vi "PP Template.vi"() -> ()   [LabVIEW 2011, in "Messenging.lvlib" / "PP Template.lvclass"]
uses:
  PP Template.lvclass
  Parallel Process.lvclass
  Interprocess Messenger/TextVarientMessage/MSG.lvclass
  Interprocess Messenger/Receiver/MGR (Receive type).lvclass
  ObserverRegister/ObserverRegistry.lvclass
  Interprocess Messenger/TextVarientMessage/Write (no data).vi
  Interprocess Messenger/TextVarientMessage/Write VarMessage.vi
  Interprocess Messenger/VarMessage/VarMessage.lvclass
  Interprocess Messenger/TextVarientMessage/Extract Text (static).vi
panel:
  out "date/time string":string
  in  "Startup Message":refnum<class "MSG.lvclass">
  # "QueueMessenger Based"
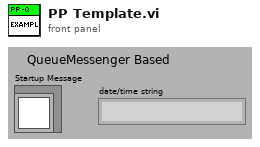
[diagram p1: front panel]
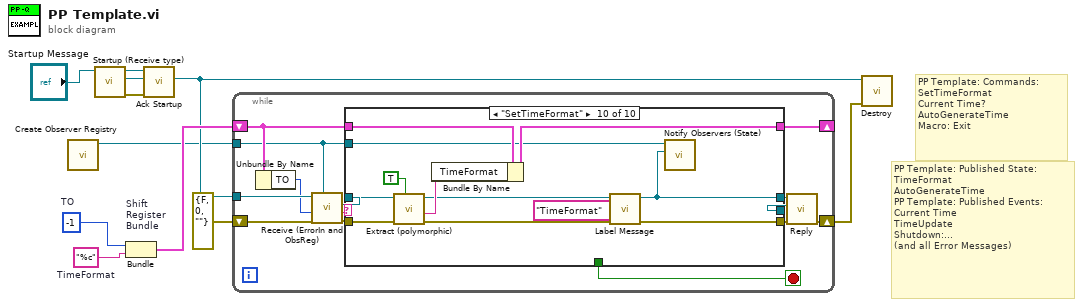
[diagram p0: block diagram]
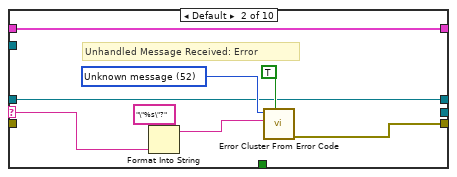
[diagram p3: hidden frame]
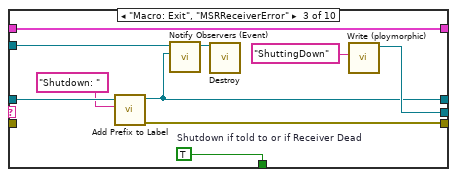
[diagram p4: hidden frame]
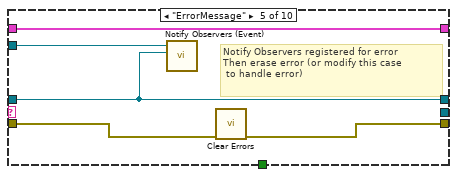
[diagram p6: hidden frame]
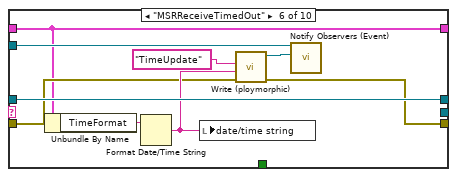
[diagram p7: hidden frame]
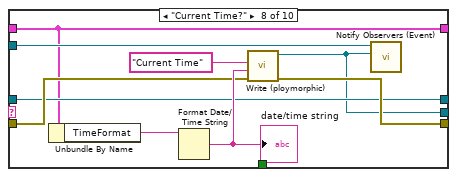
[diagram p9: hidden frame]
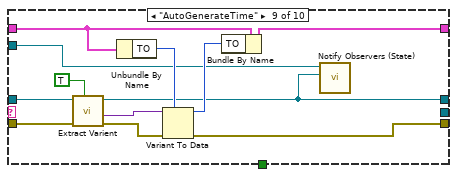
[diagram p10: hidden frame]
diagram:
  w3 = "%c"  # TimeFormat
  w8 = -1  # TO
  # "PP Template: Published State:\nTimeFormat\nAutoGenerateTime\nPP Template: Published Events:\nCurrent Time\nTimeUpdate\nShutdown:...\n(and all Error Messages)"
  # "PP Template: Commands:\nSetTimeFormat\nCurrent Time?\nAutoGenerateTime\nMacro: Exit"
  n1 = call "Create Observer Registry.vi"() -> ("ObsReg"=w2:refnum<class "ObserverRegistry.lvclass">)  [unwired: 1 in, 10 out]
  n2 = call "Startup (Receive type).vi"("Startup Message"="Startup Message") -> ("error out"=w5:errorcluster, "Command Messenger out"=w6:refnum<class "MGR (Receive type).lvclass">, "Starup Message"=w11:refnum<class "MSG.lvclass">)  [unwired: 1 in, 7 out]
  n3 = Bundle "Shift\nRegister\nBundle"("TO"=w8, "TimeFormat"=w3) -> (w7:cluster{"TO":i32, "TimeFormat":string})  [unwired: 1 out]
  n4 = call "Ack Startup.vi"("error in"=w5, "Command Messenger"=w6, "Starup Message"=w11) -> ("Command Messenger"=w4:refnum<class "MGR (Receive type).lvclass">)  [unwired: 3 in, 5 out]
  n5 = while {
    shift-right: [w23] -> w9
    shift-left: errorcluster {"status"=FALSE, "code"=0, "source"=""} ("error out") -> [w15]
    shift-right: [w20] -> _
    shift-left: w7 -> [w19]
    tunnel: w4 -> [w14]
    tunnel: w2 -> [w13]
    stop <- w21 stop-if-true
    n6 = Unbundle By Name(w19) -> ("TO"=w12:i32)
    n7 = call-dynamic "Receive (ErrorIn and ObsReg).vi"("ObserverRegistry in"=w13, "error in (no error)"=w15, "timeout in ms (-1)"=w12, "MGR in"=w14) -> ("error out"=w16:errorcluster, "Label"=w17:string, "Message"=w18:refnum<class "MSG.lvclass">)  [unwired: 5 out]
    n8 = case shown="\"SetTimeFormat\"" w17 {
      selector: w17 -> [_ w36 _ _ _ _ _ _ _ _]
      tunnel: [w27 w29 w37 w48 w50 w60 w64 w75 w81 w89] -> w22
      tunnel: [w26 w30 w38 w47 w52 w63 w65 w72 w78 w91] -> w25
      tunnel: [_ _ w41 _ _ _ _ w70 _ _] -> w24
      tunnel: [_ _ w45 _ _ _ _ _ _ _] -> w21
      tunnel: [w28 w31 w46 w49 w54 w56 w66 w68 w84 w97] -> w20
      tunnel: w19 -> [w28 w31 w46 w49 w54 w56 w66 w68 w86 w99]
      tunnel: w18 -> [w26 w30 w40 w47 w52 w63 w65 w72 w80 w98]
      tunnel: w16 -> [w27 _ _ w48 w51 w61 w64 w73 w79 w95]
      tunnel: w13 -> [_ _ w43 _ w53 w59 _ w71 w77 w94]
      frame "------- Core (don't modify) --------" {
        # "Core Cases for template"
      }
      frame Default {
        w33 = 52 items=["No error", "Argument error", "Memory is full", "Out of zone", "End of file", "File already open", "Generic file I/O error", "File not found", "File permission error", "Disk is full", "Duplicate path", "Too many files open", "System feature not enabled", "Resource file not found", "Cannot add resource", "Resource not found", "Image not found", "Image memory error", "Pen does not exist", "Config type invalid", "Config token not found", "Config parse error", "Config memory error", "Bad external code format", "Bad external code offset", "External code not present", "Null window", "Destroy window error", "Null menu", "Print aborted", "Bad print record", "Print driver error", "Windows error during printing", "Memory error during printing", "Print dialog error", "Generic print error", "Invalid device refnum", "Device not found", "Device parameter error", "Device unit error", "Cannot open device", "Device call aborted", "Generic error", "Cancelled by user", "Object ID too low", "Object ID too high", "Object not in heap", "Unknown heap", "Unknown object (invalid DefProc)", "Unknown object (DefProc not in table)", "Message out of range", "Invalid (null) method", "Unknown message", "Manager call not supported", "Bad address", "Network operation in progress", "Network operation timed out", "Connection is busy", "Network attribute not supported", "Network error", "Address in use", "System out of memory", "Connection aborted", "Connection refused", "Not connected", "Already connected", "Connection closed", "Initialization error (interapplication manager)", "Bad occurrence", "Wait on unbound occurrence handler", "Occurrence queue overflow", "Datalog type conflict", "Unused", "Unrecognized type (interapplication manager)", "Memory corrupt", "Failed to make temporary DLL", "Old CIN version", "Drag socket not found", "Failed to load drop-object", "Failed to register OLE object", "Failed to release OLE object", "Format specifier type mismatch", "Unknown format specifier", "Too few format specifiers", "Too many format specifiers", "Scan failed", "Newer CIN version", "Error converting to variant", "Runtime menu error", "Password tampered", "Variant attribute not found", "Incompatible variant data type", "Event data is not available", "Event Store is not present", "Occurrence is not found", "Event Queue is not created", "Event info is not available", "Refnum passed is NULL", "Error retrieving Class GUID", "Error retrieving CoClass GUID", "Error retrieving TypeLib GUID.", "Bad built application magic bytes.", "Specific driver is different from the specific driver associated with the Logical Name.", "There is no session opened to the class driver.", "Max Error", "MAX - Error with config objects", "MAX - Error loading configuration", "MAX - Group not supported"]
        # "Unhandled Message Received: Error"
        n9 = Format Into String(format string="\"%s\"?", w36) -> (resulting string=w34:string)  [unwired: 2 in, 1 out]
        n10 = call <vilib>:"Error Cluster From Error Code.vi"("show call chain? (False)"=TRUE, "error message (\"\")"=w34, "error code (0)"=w33) -> ("error out"=w29:errorcluster)  [unwired: 1 in, 5 out]
      }
      frame "Macro: Exit", "MSRReceiverError" {
        w45 = TRUE  # Shutdown if told to or if Receiver Dead
        n11 = call-dynamic "Add Prefix to Label.vi"("Prefix to add"="Shutdown: ", "Message"=w40) -> ("error out"=w37:errorcluster, "Message"=w38:refnum<class "MSG.lvclass">)  [unwired: 1 in, 7 out]
        n12 = call "Notify Observers (Event).vi"("Message"=w38, "ObserverRegistry in"=w43) -> ("ObserverRegistry out"=w44:refnum<class "ObserverRegistry.lvclass">)  [unwired: 1 in, 8 out]
        n13 = call "Destroy.vi"("ObserverRegistry.lvclass in"=w44) -> ()  [unwired: 1 in, 10 out]
        n14 = call-poly "Write (ploymorphic).vi"("Label"="ShuttingDown") -> ("Message"=w41:refnum<class "MSG.lvclass">)  [unwired: 1 in, 9 out]
      }
      frame "-------- Core (modify to suit) -----" {
        # "Core Cases for template"
      }
      frame "ErrorMessage" {
        # "Notify Observers registered for error\nThen erase error (or modify this case\n to handle error)"
        n15 = call "Notify Observers (Event).vi"("Message"=w52, "ObserverRegistry in"=w53) -> ()  [unwired: 1 in, 9 out]
        n16 = call <vilib>:"Clear Errors.vi"("error in (no error)"=w51) -> ("error out"=w50:errorcluster)  [unwired: 6 out]
      }
      frame "MSRReceiveTimedOut" {
        n17 = Unbundle By Name(w56) -> ("TimeFormat"=w55:string)
        n18 = Format Date/Time String(time format string (%c)=w55) -> (date/time string=w62:string)  [unwired: 2 out]
        n19 = local write "date/time string"(w62) -> ()
        n20 = call-poly "Write (ploymorphic).vi"("error in (no error)"=w61, "Varient"=w62, "Label"="TimeUpdate") -> ("error out"=w60:errorcluster, "Message"=w58:refnum<class "VarMessage.lvclass">)  [unwired: 7 out]
        n21 = call "Notify Observers (Event).vi"("Message"=w58, "ObserverRegistry in"=w59) -> ()  [unwired: 1 in, 9 out]
      }
      frame "-------- Example --------" {
        # "Example Cases: replace when using template"
      }
      frame "Current Time?" {
        n22 = Unbundle By Name(w68) -> ("TimeFormat"=w67:string)
        n23 = Format Date/Time String(time format string (%c)=w67) -> (date/time string=w74:string)  [unwired: 2 out]
        "date/time string" <- w74
        n24 = call-poly "Write (ploymorphic).vi"("error in (no error)"=w73, "Varient"=w74, "Label"="Current Time") -> ("error out"=w75:errorcluster, "Message"=w70:refnum<class "VarMessage.lvclass">)  [unwired: 7 out]
        n25 = call "Notify Observers (Event).vi"("Message"=w70, "ObserverRegistry in"=w71) -> ()  [unwired: 1 in, 9 out]
      }
      frame "AutoGenerateTime" {
        n26 = call-dynamic "Extract Varient.vi"("Copy"=TRUE, "error in (no error)"=w79, "Message"=w80) -> ("error out"=w82:errorcluster, "Varient"=w87:variant, "Message"=w78:refnum<class "MSG.lvclass">)  [unwired: 6 out]
        n27 = Unbundle By Name(w86) -> ("TO"=w85:i32)
        n28 = Variant To Data(error in=w82, type=w85, Variant=w87) -> (data=w83:i32, error out=w81:errorcluster)
        n29 = Bundle By Name(cluster=w86, "TO"=w83) -> (w84:cluster{"TO":i32, "TimeFormat":string})
        n30 = call "Notify Observers (State).vi"("State Message"=w78, "ObserverRegistry in"=w77) -> ()  [unwired: 1 in, 9 out]
      }
      frame "SetTimeFormat" {
        n31 = call-poly "Extract (polymorphic).vi"("Copy"=TRUE, "error in (no error)"=w95, "TextMessage in"=w98) -> ("error out"=w90:errorcluster, "Text"=w96:string, "TextMessage out"=w92:refnum<class "MSG.lvclass">)  [unwired: 6 out]
        n32 = Bundle By Name(cluster=w99, "TimeFormat"=w96) -> (w97:cluster{"TO":i32, "TimeFormat":string})
        n33 = call-dynamic "Label Message.vi"("error in (no error)"=w90, "Label"="TimeFormat", "Message"=w92) -> ("error out"=w89:errorcluster, "Message"=w91:refnum<class "MSG.lvclass">)  [unwired: 7 out]
        n34 = call "Notify Observers (State).vi"("State Message"=w91, "ObserverRegistry in"=w94) -> ()  [unwired: 1 in, 9 out]
      }
    }
    n35 = call-dynamic "Reply.vi"("error in (no error)"=w22, "Reply"=w24, "Message to Reply to"=w25) -> ("error out"=w23:errorcluster)  [unwired: 8 out]
  }
  n36 = call-dynamic "Destroy.vi"("error in (no error)"=w9, "Messenger in"=w4) -> ()  [unwired: 10 out]
